vi "degC to degF.vi"(11 "degreesC":dbl) -> (3 "degreesF":dbl)   [LabVIEW 2020]
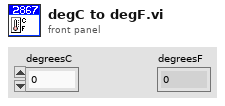
[diagram p1: front panel]
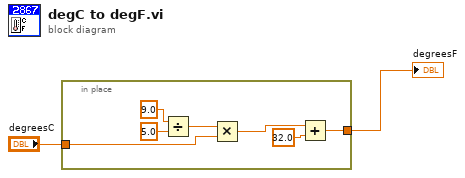
[diagram p0: block diagram]
diagram:
  n1 = in-place {
    in-place-border: "degreesC" -> [w9]
    in-place-border: [w6] -> w2
    n2 = Divide(x=9.0, y=5.0) -> (x/y=w4:dbl)
    n3 = Multiply(x=w4, y=w9) -> (x*y=w7:dbl)
    n4 = Add(x=w7, y=32.0) -> (x+y=w6:dbl)
  }
  "degreesF" <- w2
